vi "LLM_Stream.vi"() -> ()   [LabVIEW 2018]
doc: "This example demonstrates how to use OpenVINO to infer DeepSeek in LabVIEW to enable real-time streaming, processing, and display of data (e.g., text)."
uses:
  vi.lib/VIRobotics/OpenVINO_GenAI/LLMPipeline/Generate_With_Queue.vi
  vi.lib/VIRobotics/OpenVINO_GenAI/LLMPipeline/LLMPipeline.lvclass
panel:
  in  "device_name":string(combo)="CPU"
  in  "model_folder":path=path "D:/code/llm/deepseek/Deepseek-R1-1.5B-Instruct-int4-ov"
  in  "Prompt":string
  in  "send":bool
  in  "stop":bool
  out "Dialog":string
  # "Overview: This example demonstrates how to use OpenVINO to infer  DeepSeek in LabVIEW to enable real-time streaming, processing, and display of data (e.g., text). \nRequirements: Windows.\nInstructions: \n1.Download model.Select the model folder to use.\n2.Run the VI.\n3.Enter the prompt keywords.Then click Send."
  # "LLM Stream Example for LabVIEW"
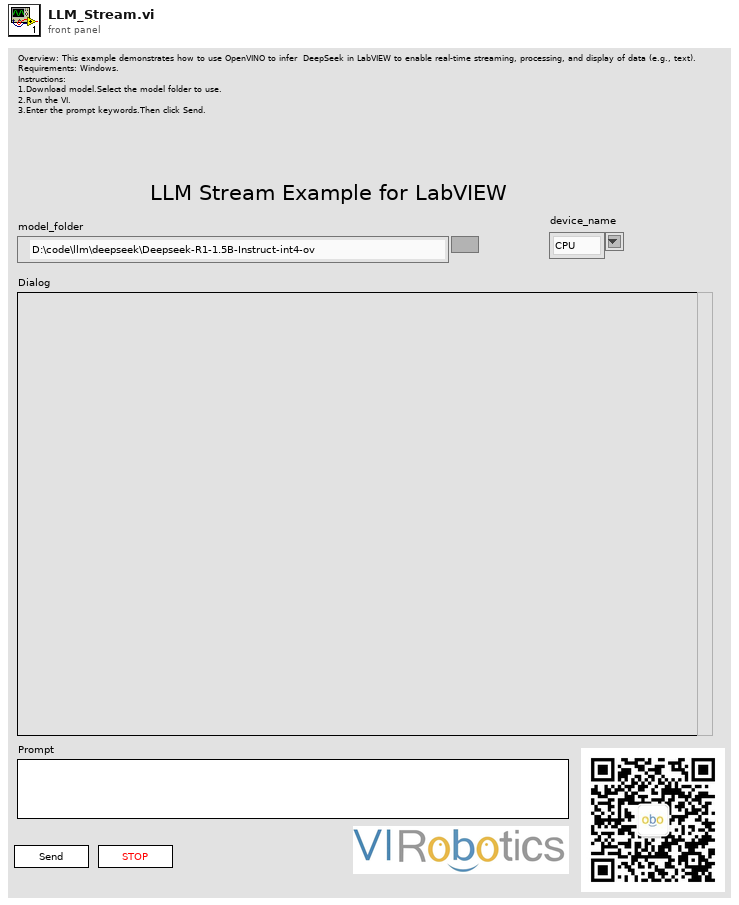
[diagram p1: front panel]
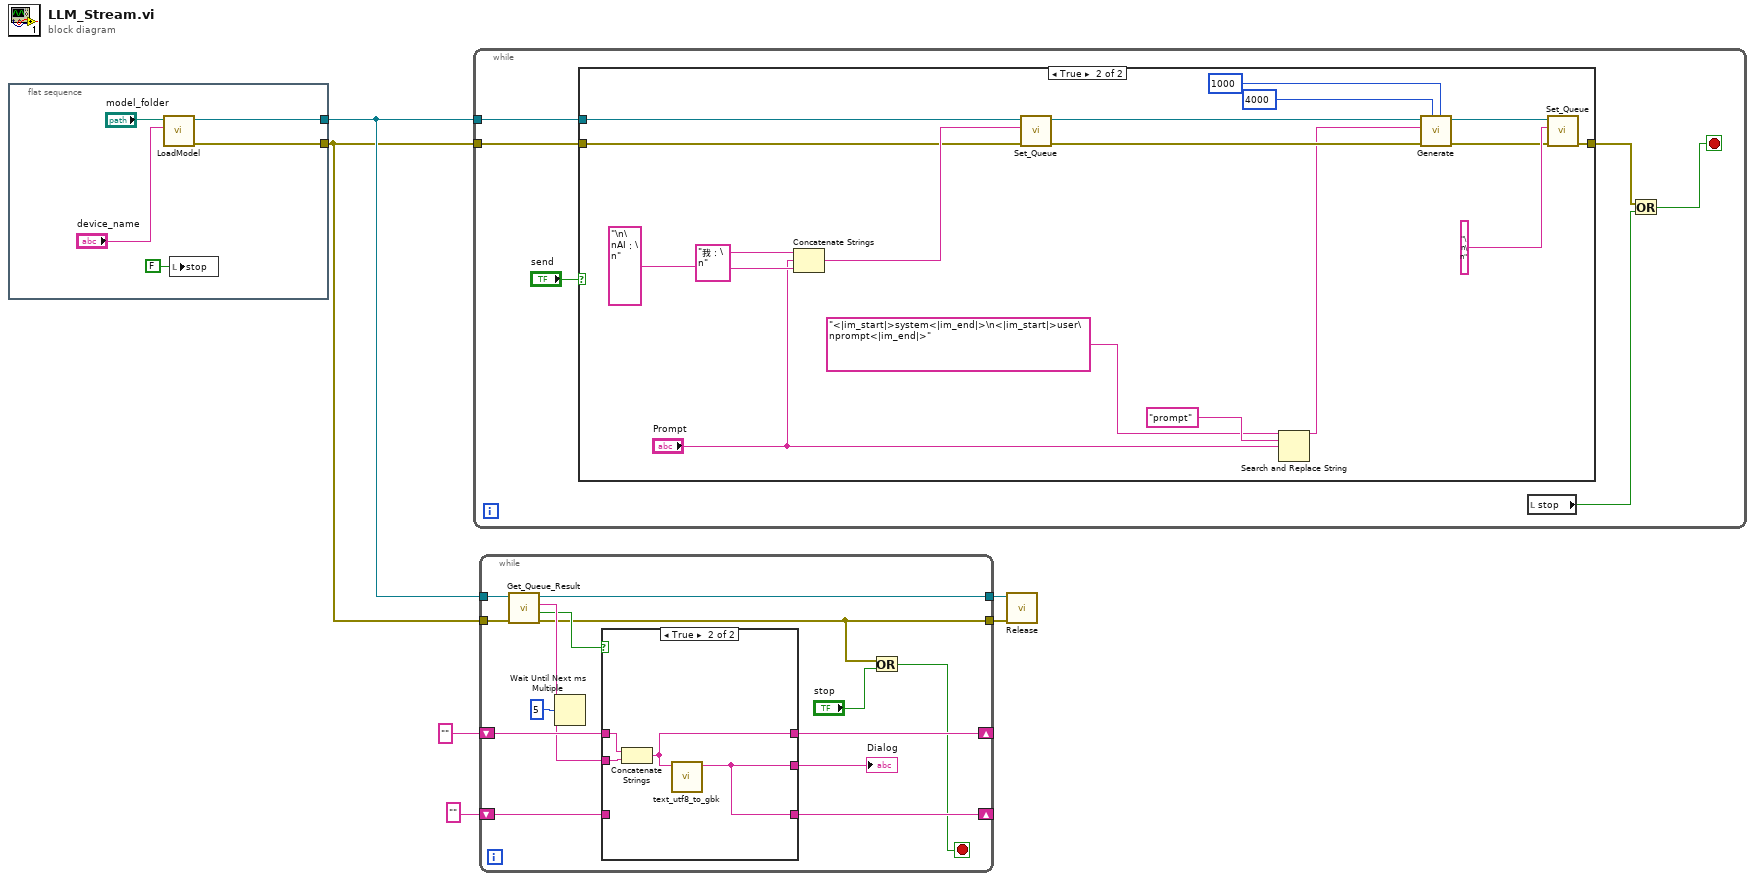
[diagram p0: block diagram]
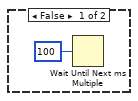
[diagram p2: hidden frame]
diagram:
  n1 = flat-sequence {
    tunnel: [w9] -> w4
    tunnel: [w8] -> w2
    frame #0 {
      n2 = call "LoadModel.vi"("device"="device_name", "path"="model_folder") -> ("error out"=w8:errorcluster, "LLMPipeline out"=w9:refnum<class "LLMPipeline.lvclass">)  [unwired: 8 in]
      n3 = local write "stop"(FALSE ("stop")) -> ()
    }
  }
  n4 = while {
    tunnel: w4 -> [w16]
    tunnel: w2 -> [w15]
    stop <- w12 stop-if-true
    n5 = case shown="True" "send" {
      tunnel: w16 -> [_ w30]
      tunnel: w15 -> [_ w27]
      tunnel: [_ w26] -> w14
      frame False {
        n6 = Wait Until Next ms Multiple(millisecond multiple=u32 100) -> ()  [unwired: 1 out]
      }
      frame True {
        n7 = Concatenate Strings("我：\n" ("string"), "Prompt", "\n\nAI：\n" ("string")) -> (w28:string)
        n8 = call "Set_Queue.vi"("error in (no error)"=w27, "text"=w28, "LLMPipeline in"=w30) -> ("error out"=w23:errorcluster, "LLMPipeline out"=w24:refnum<class "LLMPipeline.lvclass">)  [unwired: 7 in]
        n9 = Search and Replace String(input string="<|im_start|>system<|im_end|>\n<|im_start|>user\nprompt<|im_end|>", search string="prompt", replace string="Prompt") -> (result string=w19:string)  [unwired: 5 in, 3 out]
        n10 = call-poly "Generate.vi"("max_length"=1000, "max_new_tokens"=4000, "error in (no error)"=w23, "prompt"=w19, "LLMPipeline in"=w24) -> ("error out"=w22:errorcluster, "LLMPipeline out"=w25:refnum<class "LLMPipeline.lvclass">)  [unwired: 4 in, 1 out]
        n11 = call "Set_Queue.vi"("error in (no error)"=w22, "text"="\n\n" ("text_gbk"), "LLMPipeline in"=w25) -> ("error out"=w26:errorcluster)  [unwired: 7 in, 1 out]
      }
    }
    n12 = local read "stop"() -> (w13:bool)
    n13 = Or(x=w14, y=w13) -> (x .or. y?=w12:bool)
  }
  n14 = while {
    shift-right: [w47] -> _
    shift-left: "" -> [w49]
    shift-right: [w44] -> _
    shift-left: "" -> [w45]
    tunnel: w4 -> [w41]
    tunnel: [w40] -> w3
    tunnel: w2 -> [w39]
    tunnel: [w36] -> w1
    stop <- w37 stop-if-true
    n15 = call "Get_Queue_Result.vi"("error in (no error)"=w39, "LLMPipeline in"=w41) -> ("error out"=w36:errorcluster, "valid"=w42:bool, "text_out"=w43:string, "LLMPipeline out"=w40:refnum<class "LLMPipeline.lvclass">)  [unwired: 6 in]
    n16 = Wait Until Next ms Multiple(millisecond multiple=u32 5) -> ()  [unwired: 1 out]
    n17 = case shown="True" w42 {
      tunnel: w49 -> [w51 w55]
      tunnel: [w51 w53] -> w47
      tunnel: [w50 w52] -> w46
      tunnel: w43 -> [_ w54]
      tunnel: w45 -> [w50 _]
      tunnel: [w50 w52] -> w44
      frame False {
      }
      frame True {
        n18 = Concatenate Strings(w55, w54) -> (w53:string)
        n19 = call "text_utf8_to_gbk.vi"("text_utf8"=w53) -> ("text_gbk"=w52:string)  [unwired: 9 in, 1 out]
      }
    }
    "Dialog" <- w46
    n20 = Or(x=w36, y="stop") -> (x .or. y?=w37:bool)
  }
  n21 = call "Release.vi"("error in (no error)"=w1, "LLMPipeline in"=w3) -> ()  [unwired: 8 in, 2 out]
